vi "CameraSetTrigger.vi"(8 "error in (no error)":errorcluster, 10 "external?":bool=TRUE, 11 "IMAQdx in":refnum<class "IMAQdx_Flea3_Firewire.lvclass">) -> (0 "error out":errorcluster, 2 "attribs":variant[](array[variant]), 3 "IMAQdx out":refnum<class "IMAQdx_Flea3_Firewire.lvclass">)   [LabVIEW 2012, in "IMAQdx_Flea3_Firewire.lvclass"]
uses:
  <userlib>/bias2/classes/IMAQdx_Flea3_Firewire/IMAQdx_Flea3_Firewire.lvclass
  <userlib>/bias2/classes/IMAQdx_Flea3_Firewire/IMAQdx_Flea3_Firewire.lvclass/IMAQdx_Flea3_Firewire.ctl
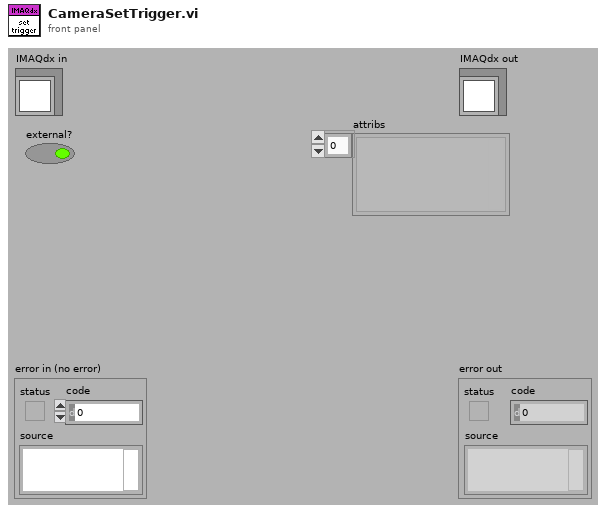
[diagram p1: front panel]
types:
  T1 = typedef "IMAQdx.ctl" = refnum<k21>
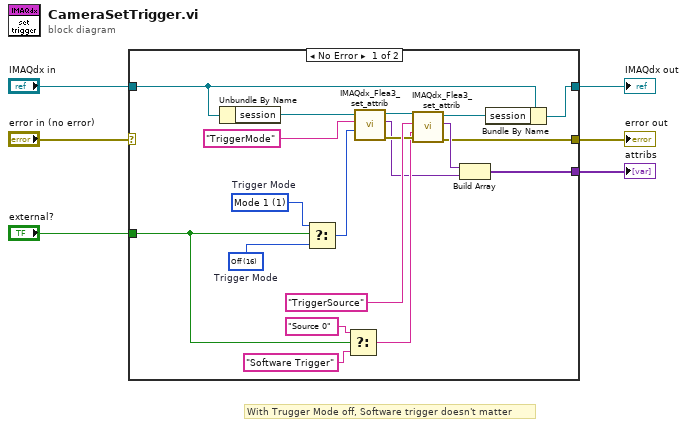
[diagram p0: block diagram]
diagram:
  # "With Trugger Mode off, Software trigger doesn't matter"
  n1 = case shown="No Error" "error in (no error)" {
    selector: "error in (no error)" -> [_ w27]
    tunnel: [w13 w27] -> w5
    tunnel: [w17 w26] -> w3
    tunnel: "IMAQdx in" -> [w18 w26]
    tunnel: [w12 _] -> w2
    tunnel: "external?" -> [w10 _]
    frame No Error {
      w7 = u32 16 items=["Mode 0"=0, "Mode 1"=1, "Mode 3"=3, "Mode 14"=14, "Mode 15"=15, "Off"=16]  # Trigger Mode
      w9 = u32 1 items=["Mode 0"=0, "Mode 1"=1, "Mode 3"=3, "Mode 14"=14, "Mode 15"=15, "Off"=16]  # Trigger Mode
      n2 = Unbundle By Name(w18) -> ("session"=w11:refnum<k21>)
      n3 = Select(t=w9, s=w10, f=w7) -> (s? t:f=w8:u32)
      n4 = Select(t="Source 0", s=w10, f="Software Trigger") -> (s? t:f=w19:string)
      n5 = call <userlib>:"IMAQdx_Flea3_set_attrib.vi"("value"=w8, "attribute"="TriggerMode" ("ActiveAttribute"), "IMAQdx in"=w11) -> ("error out"=w22:errorcluster, "attrib out"=w14:variant, "IMAQdx out"=w25:T1)  [unwired: 2 in]
      n6 = call <userlib>:"IMAQdx_Flea3_set_attrib.vi"("error in"=w22, "value"=w19, "attribute"="TriggerSource" ("ActiveAttribute"), "IMAQdx in"=w25) -> ("error out"=w13:errorcluster, "attrib out"=w15:variant, "IMAQdx out"=w16:T1)  [unwired: 1 in]
      n7 = Build Array(w15, w14) -> (w12:variant[])
      n8 = Bundle By Name(cluster=w18, "session"=w16) -> (w17:refnum<class "IMAQdx_Flea3_Firewire.lvclass">)
    }
    frame Error {
    }
  }
  "error out" <- w5
  "IMAQdx out" <- w3
  "attribs" <- w2
